vi "总磷总氮版本号读取.vi"(8 "Error in":errorcluster caption="Error in (no error)", 11 "Slave ID":u8=3) -> (0 "error out":errorcluster, 3 "固件版本号":string)   [LabVIEW 2016, in "斯坦道氨氮.lvlib"]
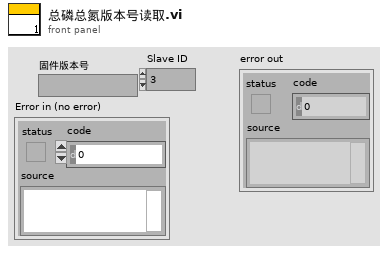
[diagram p1: front panel]
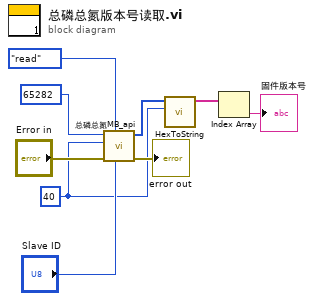
[diagram p0: block diagram]
diagram:
  w1 = u16 40 ("quantity")
  n1 = call "总磷总氮MB_api.vi"("Slave ID"="Slave ID", "STEP"=enum16{"open", "read", "write", "close"}."read", "Error in"="Error in", "quantity"=w1, "starting address"=u16 65282) -> ("error out"=→"error out":errorcluster, "Registers"=w4:u16[])  [unwired: 4 in, 1 out]
  n2 = call "HexToString.vi"("字符个数"=w1, "数组"=w4) -> ("STRING"=w3:string[])  [unwired: 9 in]
  n3 = Index Array(array=w3) -> (element=→"固件版本号":string)  [unwired: 1 in]
